vi "After Read.vi"(8 "error in":errorcluster, 9 "State In":variant, 10 "Compiled Settings":variant, 11 "Custom Device API in":refnum<class "Custom Device API.lvclass">) -> (0 "error out":errorcluster, 1 "State Out":variant, 3 "Custom Device API out":refnum<class "Custom Device API.lvclass">)   [LabVIEW 2026, in "SystemMonitor Test Hooks.lvlib"]
uses:
  SystemMonitor Test Hooks.lvlib
  <userlib>/Custom Device Interfaces_v1.lvlibp/CustomDeviceAPI/Custom Device API.lvclass
  Shared/Compiled.Settings.ctl
  Shared/CustomDeviceSettings.ctl
  Shared/ChannelGroups.ctl
  Shared/GroupedChannelRefs.ctl
  Shared/GroupSettings.ctl
  Shared/GroupedChannel.ctl
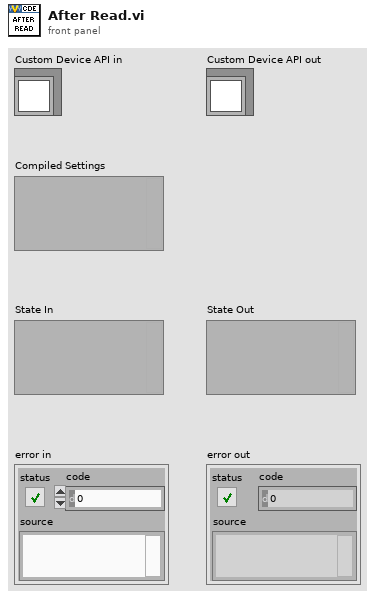
[diagram p1: front panel]
types:
  T1 = typedef "Compiled.Settings.ctl" = cluster{"SystemMonitor":T2, "Channel Groups":T3}
  T2 = typedef "CustomDeviceSettings.ctl" = cluster{"Name":string, "Properties":cluster{"Update Rate (Hz)":dbl, "TargetOS":string, "TargetRate":dbl}, "Sections":cluster{"CPUOverall[]":cluster{"Name":string, "Channels":cluster{"AverageType[]":cluster{"Name":string, "DefaultValue":dbl, "Units":string, "GroupName":string, "Type":string, "Faultable":bool, "Scalable":bool, "ChannelDataReference":i32, "GroupIndex":i32}[], "MaximumType[]":cluster{"Name":string, "DefaultValue":dbl, "Units":string, "GroupName":string, "Type":string, "Faultable":bool, "Scalable":bool, "ChannelDataReference":i32, "GroupIndex":i32}[]}}[], "MemoryUsage[]":cluster{"Name":string, "Channels":cluster{"TotalMemoryType[]":cluster{"Name":string, "DefaultValue":dbl, "Units":string, "GroupName":string, "Type":string, "Faultable":bool, "Scalable":bool, "ChannelDataReference":i32, "GroupIndex":i32}[], "AvailableType[]":cluster{"Name":string, "DefaultValue":dbl, "Units":string, "GroupName":string, "Type":string, "Faultable":bool, "Scalable":bool, "ChannelDataReference":i32, "GroupIndex":i32}[]}}[], "CPU[]":cluster{"Name":string, "Channels":cluster{"TotalType[]":cluster{"Name":string, "DefaultValue":dbl, "Units":string, "GroupName":string, "Type":string, "Faultable":bool, "Scalable":bool, "ChannelDataReference":i32, "GroupIndex":i32}[], "TimeCriticalType[]":cluster{"Name":string, "DefaultValue":dbl, "Units":string, "GroupName":string, "Type":string, "Faultable":bool, "Scalable":bool, "ChannelDataReference":i32, "GroupIndex":i32}[], "TimedStructuresType[]":cluster{"Name":string, "DefaultValue":dbl, "Units":string, "GroupName":string, "Type":string, "Faultable":bool, "Scalable":bool, "ChannelDataReference":i32, "GroupIndex":i32}[], "HighType[]":cluster{"Name":string, "DefaultValue":dbl, "Units":string, "GroupName":string, "Type":string, "Faultable":bool, "Scalable":bool, "ChannelDataReference":i32, "GroupIndex":i32}[], "AboveNormalType[]":cluster{"Name":string, "DefaultValue":dbl, "Units":string, "GroupName":string, "Type":string, "Faultable":bool, "Scalable":bool, "ChannelDataReference":i32, "GroupIndex":i32}[], "NormalType[]":cluster{"Name":string, "DefaultValue":dbl, "Units":string, "GroupName":string, "Type":string, "Faultable":bool, "Scalable":bool, "ChannelDataReference":i32, "GroupIndex":i32}[], "BackgroundType[]":cluster{"Name":string, "DefaultValue":dbl, "Units":string, "GroupName":string, "Type":string, "Faultable":bool, "Scalable":bool, "ChannelDataReference":i32, "GroupIndex":i32}[], "IdleType[]":cluster{"Name":string, "DefaultValue":dbl, "Units":string, "GroupName":string, "Type":string, "Faultable":bool, "Scalable":bool, "ChannelDataReference":i32, "GroupIndex":i32}[], "ISRType[]":cluster{"Name":string, "DefaultValue":dbl, "Units":string, "GroupName":string, "Type":string, "Faultable":bool, "Scalable":bool, "ChannelDataReference":i32, "GroupIndex":i32}[]}}[]}}
  T3 = typedef "ChannelGroups.ctl" = cluster{"Channel Refs":T4, "Group Settings":T5[]}
  T4 = typedef "GroupedChannelRefs.ctl" = cluster{"Read":cluster{"Refs":cluster{"Data Reference":i32, "Offset":u64, "Length":u64}[], "Values":dbl[]}[], "Write":cluster{"Refs":cluster{"Data Reference":i32, "Offset":u64, "Length":u64}[], "Values":dbl[]}[], "ReadWrite":cluster{"Refs":i32[], "Values":dbl[], "Reset Values":dbl[]}[], "LUT":variant}
  T5 = typedef "GroupSettings.ctl" = cluster{"Name":string, "Type":enum16{"Output/Write", "Input/Read", "Input/ReadWrite"}, "Channel Settings":T6[]}
  T6 = typedef "GroupedChannel.ctl" = cluster{"Name":string, "TypeName":string, "ChannelProperties":variant}
  T7 = cluster{"Name":string, "Channels":cluster{"AverageType[]":cluster{"Name":string, "DefaultValue":dbl, "Units":string, "GroupName":string, "Type":string, "Faultable":bool, "Scalable":bool, "ChannelDataReference":i32, "GroupIndex":i32}[], "MaximumType[]":cluster{"Name":string, "DefaultValue":dbl, "Units":string, "GroupName":string, "Type":string, "Faultable":bool, "Scalable":bool, "ChannelDataReference":i32, "GroupIndex":i32}[]}}[]
  T8 = cluster{"Name":string, "DefaultValue":dbl, "Units":string, "GroupName":string, "Type":string, "Faultable":bool, "Scalable":bool, "ChannelDataReference":i32, "GroupIndex":i32}[]
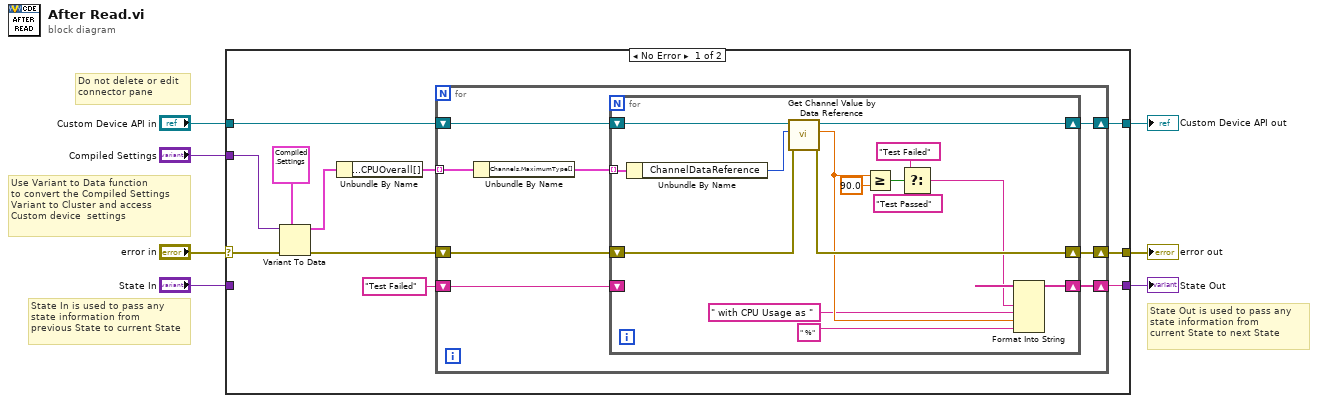
[diagram p0: block diagram]
diagram:
  # "State Out is used to pass any \nstate information from\ncurrent State to next State"
  # "State In is used to pass any \nstate information from\nprevious State to current State"
  # "Use Variant to Data function\nto convert the Compiled Settings\nVariant to Cluster and access \nCustom device  settings"
  # "Do not delete or edit \nconnector pane"
  n1 = case shown="No Error" "error in" {
    selector: "error in" -> [w16 w43]
    tunnel: [w14 w43] -> w6
    tunnel: "Custom Device API in" -> [w18 w44]
    tunnel: [w15 w44] -> w4
    tunnel: "State In" -> [_ w42]
    tunnel: [w13 w42] -> w2
    tunnel: "Compiled Settings" -> [w17 _]
    frame No Error {
      n2 = Variant To Data(error in=w16, type=T1 {"SystemMonitor"={"Name"="", "Properties"={"Update Rate (Hz)"=0.0, "TargetOS"="", "TargetRate"=0.0}, "Sections"={"CPUOverall[]"=[], "MemoryUsage[]"=[], "CPU[]"=[]}}, "Channel Groups"={"Channel Refs"={"Read"=[], "Write"=[], "ReadWrite"=[], "LUT"=variant}, "Group Settings"=[]}} ("Compiled Settings"), Variant=w17) -> (data=w11:T1, error out=w9:errorcluster)
      n3 = Unbundle By Name(w11) -> ("SystemMonitor.Sections.CPUOverall[]"=w10:T7)
      n4 = for {
        tunnel: w10 -> [w26] mode=indexing
        shift-right: [w23] -> w15
        shift-left: w18 -> [w24]
        shift-right: [w21] -> w14
        shift-left: w9 -> [w22]
        shift-right: [w20] -> w13
        shift-left: "Test Failed" -> [w19]
        n5 = Unbundle By Name(w26) -> ("Channels.MaximumType[]"=w25:T8)
        n6 = for {
          tunnel: w25 -> [w41] mode=indexing
          shift-right: [w38] -> w23
          shift-left: w24 -> [w40]
          shift-right: [w36] -> w21
          shift-left: w22 -> [w37]
          shift-right: [w28] -> w20
          shift-left: w19 -> [_]
          n7 = Unbundle By Name(w41) -> ("ChannelDataReference"=w39:i32)
          n8 = call-dynamic "Get Channel Value by Data Reference.vi"("error in"=w37, "Data Reference in"=w39, "Custom Device API in"=w40) -> ("error out"=w36:errorcluster, "Value"=w31:dbl, "Custom Device API out"=w38:refnum<class "Custom Device API.lvclass">)  [unwired: 6 in]
          n9 = Greater Or Equal?(x=w31, y=90.0) -> (x >= y?=w34:bool)
          n10 = Select(t="Test Failed", s=w34, f="Test Passed") -> (s? t:f=w27:string)
          n11 = Format Into String(w27, " with CPU Usage as " ("input 2"), w31, " %" ("input 2")) -> (resulting string=w28:string)  [unwired: 3 in, 1 out]
        }
      }
    }
    frame Error {
    }
  }
  "Custom Device API out" <- w4
  "error out" <- w6
  "State Out" <- w2
